vi "SnoTestDoubleSolenoid.vi"(6 "Button 10":bool, 7 "Button 11":bool, 9 "Button 7":bool, 10 "Button 6":bool, 11 "refnum name":string) -> ()   [LabVIEW 2013]
uses:
  <vilib>/Rock Robotics/WPI/Solenoid/WPI_SolenoidValue.ctl
  <vilib>/Rock Robotics/WPI/Solenoid/WPI_SolenoidSetEnum.vi
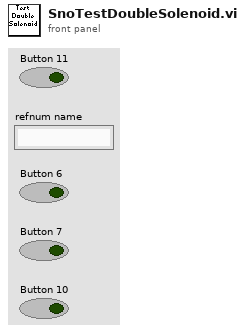
[diagram p1: front panel]
types:
  T1 = typedef "WPI_SolenoidValue.ctl" = enum16{"Off", "On", "Forward", "Reverse"}
  T2 = typedef "WPI_SolenoidDevRef.ctl" = cluster{"DevStatus":errorcluster, "Solenoid Module":T3, "Forward Solenoid Channel":T4, "Reverse Solenoid Channel":T4}
  T3 = typedef "FPGA_TypedefSolenoidModule.ctl" = enum16{"Solenoid Module 1", "Solenoid Module 2"}
  T4 = typedef "WPI_SolenoidChannel.ctl" = enum8{"Solenoid 1", "Solenoid 2", "Solenoid 3", "Solenoid 4", "Solenoid 5", "Solenoid 6", "Solenoid 7", "Solenoid 8", "Invalid"}
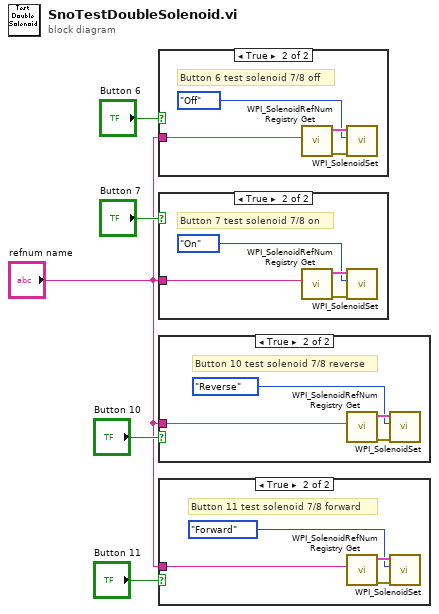
[diagram p0: block diagram]
diagram:
  n1 = case shown="True" "Button 6" {
    tunnel: "refnum name" -> [_ w6]
    frame False {
      # "Button 6 test solenoid 7/8 off"
    }
    frame True {
      # "Button 6 test solenoid 7/8 off"
      n2 = call <vilib>:"WPI_SolenoidRefNum Registry Get.vi"("refnum name"=w6) -> ("error out"=w9:errorcluster, "SolenoidDevRef"=w8:T2)  [unwired: 9 in]
      n3 = call-poly <vilib>:"WPI_SolenoidSet.vi"("error in (no error)"=w9, "Value"=WPI_SolenoidValue."Off", "SolenoidDevRef"=w8) -> ()  [unwired: 7 in, 2 out]
    }
  }
  n4 = case shown="True" "Button 7" {
    tunnel: "refnum name" -> [_ w10]
    frame False {
      # "Button 7 test solenoid 7/8 on"
    }
    frame True {
      # "Button 7 test solenoid 7/8 on"
      n5 = call <vilib>:"WPI_SolenoidRefNum Registry Get.vi"("refnum name"=w10) -> ("error out"=w13:errorcluster, "SolenoidDevRef"=w12:T2)  [unwired: 9 in]
      n6 = call-poly <vilib>:"WPI_SolenoidSet.vi"("error in (no error)"=w13, "Value"=WPI_SolenoidValue."On", "SolenoidDevRef"=w12) -> ()  [unwired: 7 in, 2 out]
    }
  }
  n7 = case shown="True" "Button 10" {
    tunnel: "refnum name" -> [_ w14]
    frame False {
      # "Button 10 test solenoid 7/8 reverse"
    }
    frame True {
      # "Button 10 test solenoid 7/8 reverse"
      n8 = call <vilib>:"WPI_SolenoidRefNum Registry Get.vi"("refnum name"=w14) -> ("error out"=w17:errorcluster, "SolenoidDevRef"=w16:T2)  [unwired: 9 in]
      n9 = call-poly <vilib>:"WPI_SolenoidSet.vi"("error in (no error)"=w17, "Value"=WPI_SolenoidValue."Reverse", "SolenoidDevRef"=w16) -> ()  [unwired: 7 in, 2 out]
    }
  }
  n10 = case shown="True" "Button 11" {
    tunnel: "refnum name" -> [_ w18]
    frame False {
      # "Button 11 test solenoid 7/8 forward"
    }
    frame True {
      # "Button 11 test solenoid 7/8 forward"
      n11 = call <vilib>:"WPI_SolenoidRefNum Registry Get.vi"("refnum name"=w18) -> ("error out"=w21:errorcluster, "SolenoidDevRef"=w20:T2)  [unwired: 9 in]
      n12 = call-poly <vilib>:"WPI_SolenoidSet.vi"("error in (no error)"=w21, "Value"=WPI_SolenoidValue."Forward", "SolenoidDevRef"=w20) -> ()  [unwired: 7 in, 2 out]
    }
  }
